vi "Telescope Init.vi"(8 "error in (no error)":errorcluster, 9 "Settings":variant, 10 "Name":string, 11 "LDT Telescope in":refnum<class "LDT Telescope.lvclass">) -> (0 "error out":errorcluster, 1 "Connect Message":string, 2 "Channel List":refnum<class "HK Item.lvclass">[](array[class]), 3 "LDT Telescope out":refnum<class "LDT Telescope.lvclass">)   [LabVIEW 2022 SP3, in "LDT Telescope.lvclass"]
uses:
  LDT Telescope.lvclass
  C:/Development/rimas/RIMAS/Telescope/Telescope.lvclass
  hk-channel-class/hk-channel-class/HK Item/HK Item.lvclass
  typedef cluster LDT Telescope Settings.ctl
  Telescope.lvclass
  LDT Telescope.lvclass/LDT Telescope.ctl
  LDT Telescope Loop.vi
  TCS/DCT-related/Common/Communication/ActiveMQ/ActiveMQBroker/ActiveMQBroker.lvclass
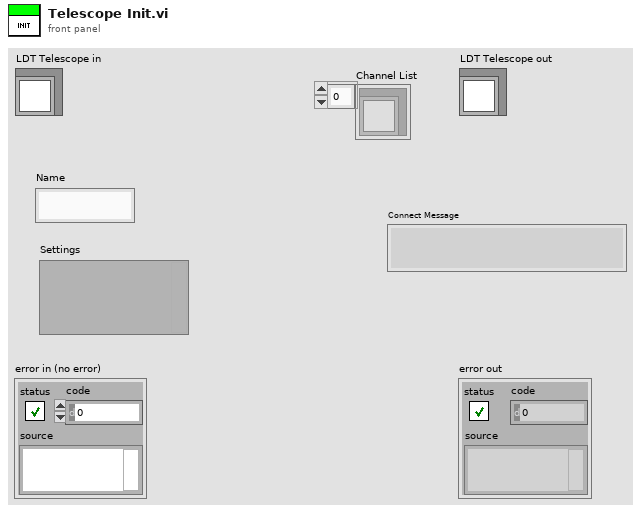
[diagram p1: front panel]
types:
  T1 = typedef "LDT Telescope.lvclass/typedef cluster LDT Telescope Settings.ctl" = cluster{"host":string, "port":string}
  T2 = enum32{"invalid app kind", "Development System", "Run Time System", "Student Edition", "Embedded LabVIEW", "Evaluation", "Custom"}
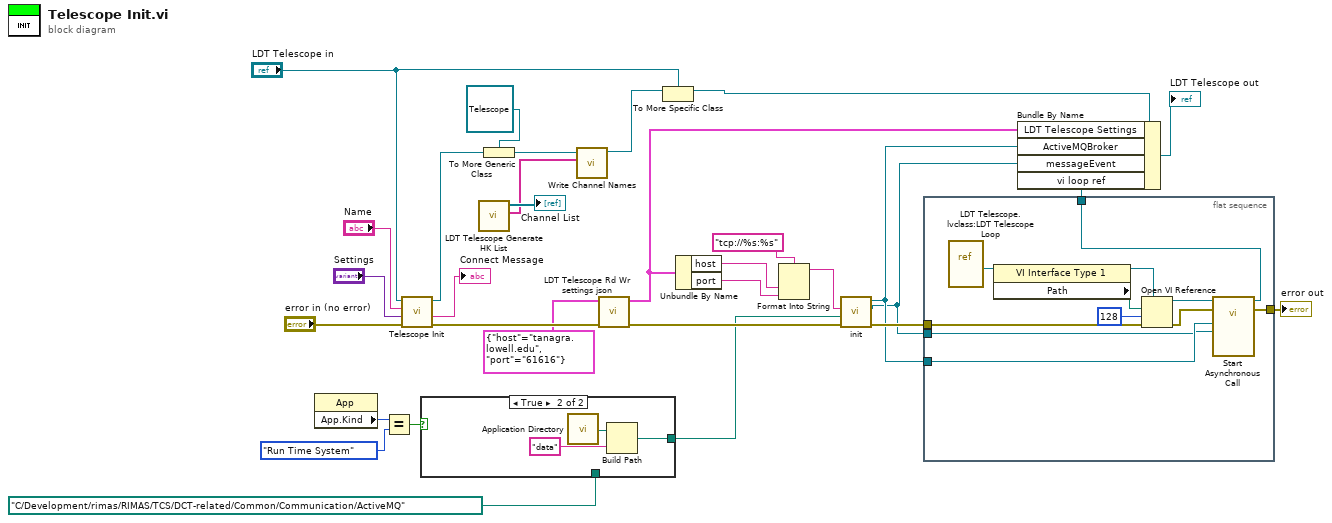
[diagram p0: block diagram]
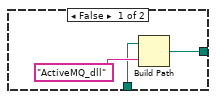
[diagram p2: hidden frame]
diagram:
  n1 = property class="App"() -> ("App.Kind"=w25:T2)  [unwired: 2 in, 2 out]
  n2 = Equal?(x=w25, y=T2."Run Time System") -> (x = y?=w23:bool)
  n3 = call-parent "Telescope Init.vi"("error in (no error)"="error in (no error)", "Settings"="Settings", "Name"="Name", "Telescope in"="LDT Telescope in") -> ("error out"=w22:errorcluster, "Connect Message"=→"Connect Message":string, "Telescope out"=w4:refnum<class "LDT Telescope.lvclass">)  [unwired: 4 in, 1 out]
  n4 = case shown="True" w23 {
    tunnel: [w33 w35] -> w15
    tunnel: path "C:/Development/rimas/RIMAS/TCS/DCT-related/Common/Communication/ActiveMQ" -> [w32 _]
    frame False {
      n5 = Build Path(base path=w32, name or relative path="ActiveMQ_dll") -> (appended path=w33:path)
    }
    frame True {
      n6 = call <vilib>:"Application Directory.vi"() -> ("Application Directory"=w37:path)
      n7 = Build Path(base path=w37, name or relative path="data") -> (appended path=w35:path)
    }
  }
  n8 = call "LDT Telescope Generate HK List.vi"() -> ("Channel Names"=w5:string[], "Channel List"=→"Channel List":refnum<class "HK Item.lvclass">[])  [unwired: 10 in]
  n9 = To More Generic Class(target class=refnum<class "Telescope.lvclass"> refnum ("Telescope.lvclass"), reference=w4) -> (generic class reference=w6:refnum<class "Telescope.lvclass">)
  n10 = call-dynamic "Write Channel Names.vi"("Channel Names"=w5, "Telescope in"=w6) -> ("Telescope out"=w2:refnum<class "Telescope.lvclass">)  [unwired: 8 in, 1 out]
  n11 = call "LDT Telescope Rd Wr settings json.vi"("error in (no error)"=w22, "LDT Telescope Settings"=T1 {"host"="tanagra.lowell.edu", "port"="61616"}) -> ("error out"=w16:errorcluster, "LDT Telescope Settings"=w19:T1)  [unwired: 8 in]
  n12 = To More Specific Class(target class="LDT Telescope in", reference=w2) -> (specific class reference=w1:refnum<class "LDT Telescope.lvclass">)  [unwired: 1 in, 1 out]
  n13 = Unbundle By Name(w19) -> ("host"=w18:string, "port"=w17:string)
  n14 = Format Into String(format string="tcp://%s:%s", w18, w17) -> (resulting string=w26:string)  [unwired: 2 in, 1 out]
  n15 = call "init.vi"("error in (no error)"=w16, "activeMQ_dll_directory"=w15, "brokerConnectionString"=w26) -> ("error out"=w14:errorcluster, "messageEvent"=w12:refnum<user-event>, "ActiveMQBroker out"=w13:refnum<class "ActiveMQBroker.lvclass">)  [unwired: 6 in]
  n16 = flat-sequence {
    tunnel: w14 -> [w45]
    tunnel: w13 -> [w41]
    tunnel: w12 -> [w40]
    tunnel: [w39] -> w11
    tunnel: [w38] -> w10
    frame #0 {
      n17 = vi-ref "LDT Telescope.lvclass:LDT Telescope Loop.vi"() -> (w48:refnum<vi>)
      n18 = property class="VI Interface Type 1"(reference=w48) -> (reference out=w43:refnum<vi>, "Path"=w47:path)  [unwired: 1 in, 1 out]
      n19 = Open VI Reference(type specifier VI Refnum (for type only)=w43, vi path=w47, options=128, error in (no error)=w45) -> (vi reference=w44:refnum<vi>, error out=w42:errorcluster)  [unwired: 2 in]
      n20 = call-by-ref "Start Asynchronous Call"(reference=w44, error in=w42, "messageEvent"=w40, "ActiveMQBroker out"=w41) -> (reference out=w38:refnum<vi>, error out=w39:errorcluster)  [unwired: 10 in]
    }
  }
  n21 = Bundle By Name(cluster=w1, "LDT Telescope Settings"=w19, "ActiveMQBroker"=w13, "messageEvent"=w12, "vi loop ref"=w10) -> (→"LDT Telescope out":refnum<class "LDT Telescope.lvclass">)
  "error out" <- w11
